vi "SOM_Globals.vi"() -> ()   [LabVIEW 2015]
panel:
  in  "Progress":refnum<vi>
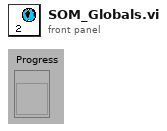
[diagram p1: front panel]
diagram:
